vi "Compute VS Channel Handle Indices.vi"(8 "error in (no error)":errorcluster, 9 "next index":i32, 11 "messages and subaddresses":T1[](array[typedef]) {"Timestamp Channel Handle" format="%.0x"; "Message Section Handle" format="%.0x"; "Parameter Channel Handles" format="%.0x"}) -> (0 "error out":errorcluster, 1 "next index out":i32, 2 "channel handles":T2[](array[typedef]) format="%.0x", 3 "messages and subaddresses out":T1[](array[typedef]) {"Timestamp Channel Handle" format="%.0x"; "Message Section Handle" format="%.0x"; "Parameter Channel Handles" format="%.0x"})   [LabVIEW 2020, in "AIM MIL-STD-1553 Engine.lvlib" / "Implementation.lvlib" / "Execution Unit.lvclass"]
uses:
  Execution Unit.lvclass
  <vilib>/NI VeriStand/Custom Device API/Custom Device Item Ref.ctl
  Custom Device/Compiled Message.ctl
  Shared/Direction.ctl
  Shared/Parameter Definition.ctl
  <vilib>/NI VeriStand/Custom Device API/Custom Device API.lvlib
  Custom Device/Custom Device.lvlib
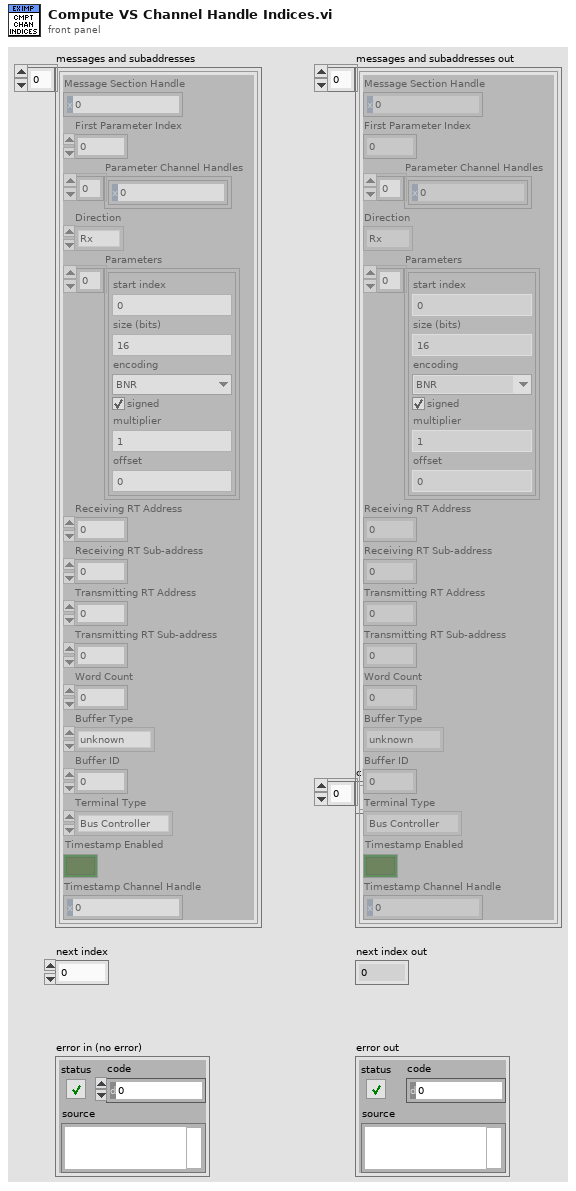
[diagram p1: front panel]
types:
  T1 = typedef "AIM MIL-STD-1553 Engine.lvlib/Custom Device.lvlib/Compiled Message.ctl" = cluster{"Message Section Handle":T2, "First Parameter Index":i32, "Parameter Channel Handles":T2[], "Direction":T3, "Parameters":T4[], "Receiving RT Address":u8, "Receiving RT Sub-address":u8, "Transmitting RT Address":u8, "Transmitting RT Sub-address":u8, "Word Count":u8, "Buffer Type":enum16{"unknown", "BC Message Buffer", "RT Message Buffer"}, "Buffer ID":u16, "Terminal Type":enum16{"Bus Controller", "Remote Terminal"}, "Timestamp Enabled":bool, "Timestamp Channel Handle":T2}
  T2 = typedef "Custom Device API.lvlib/Custom Device Item Ref.ctl" = u64
  T3 = typedef "Direction.ctl" = enum16{"Rx", "Tx"}
  T4 = typedef "Parameter Definition.ctl" = cluster{"start index":i32, "size (bits)":i32, "encoding":enum16{"BNR", "BCD", "Discrete"}, "signed":bool, "multiplier":dbl, "offset":dbl}
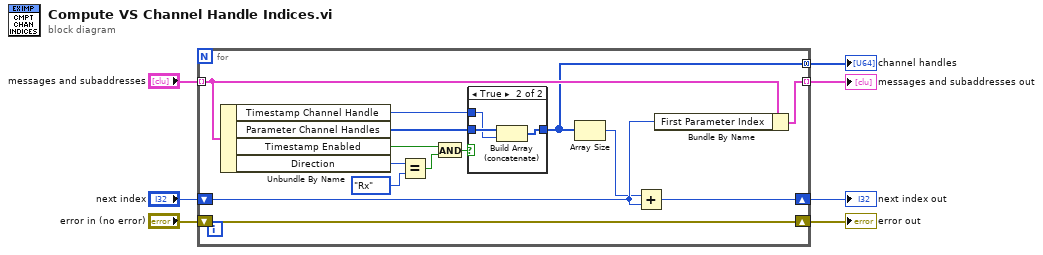
[diagram p0: block diagram]
diagram:
  n1 = for {
    tunnel: "messages and subaddresses" -> [w20] mode=indexing
    shift-right: [w21] -> w5
    shift-left: "error in (no error)" -> [w21]
    shift-right: [w19] -> w2
    shift-left: "next index" -> [w17]
    tunnel: [w18] -> w7 mode=indexing
    tunnel: [w14] -> w1 mode=concatenating
    n2 = Unbundle By Name(w20) -> ("Timestamp Channel Handle"=w15:T2, "Parameter Channel Handles"=w16:T2[], "Timestamp Enabled"=w9:bool, "Direction"=w12:T3)
    n3 = Equal?(x=w12, y=Direction."Rx" ("Direction")) -> (x = y?=w10:bool)
    n4 = And(x=w9, y=w10) -> (x .and. y?=w11:bool)
    n5 = case shown="True" w11 {
      tunnel: w16 -> [w22 w25]
      tunnel: w15 -> [_ w24]
      tunnel: [w22 w23] -> w14
      frame False {
      }
      frame True {
        n6 = Build Array (concatenate)(w25, w24) -> (w23:T2[])
      }
    }
    n7 = Array Size(array=w14) -> (size(s)=w8:i32)
    n8 = Add(x=w8, y=w17) -> (x+y=w19:i32)
    n9 = Bundle By Name(cluster=w20, "First Parameter Index"=w17) -> (w18:T1)
  }
  "channel handles" <- w1
  "messages and subaddresses out" <- w7
  "error out" <- w5
  "next index out" <- w2
